vi "HEWH OSI Calculations.vi"(8 "Error In":errorcluster, 11 "Pressure Adjusted in":T1) -> (0 "Error Out":errorcluster, 1 "Power (Watts)":dbl, 2 "Current (Amps)":dbl, 3 "Pressure Adjusted out":T1, 4 "Voltage (Volts)":dbl)   [LabVIEW 2016]
uses:
  Type Definitions/HEWH MW100 Data Cluster.ctl
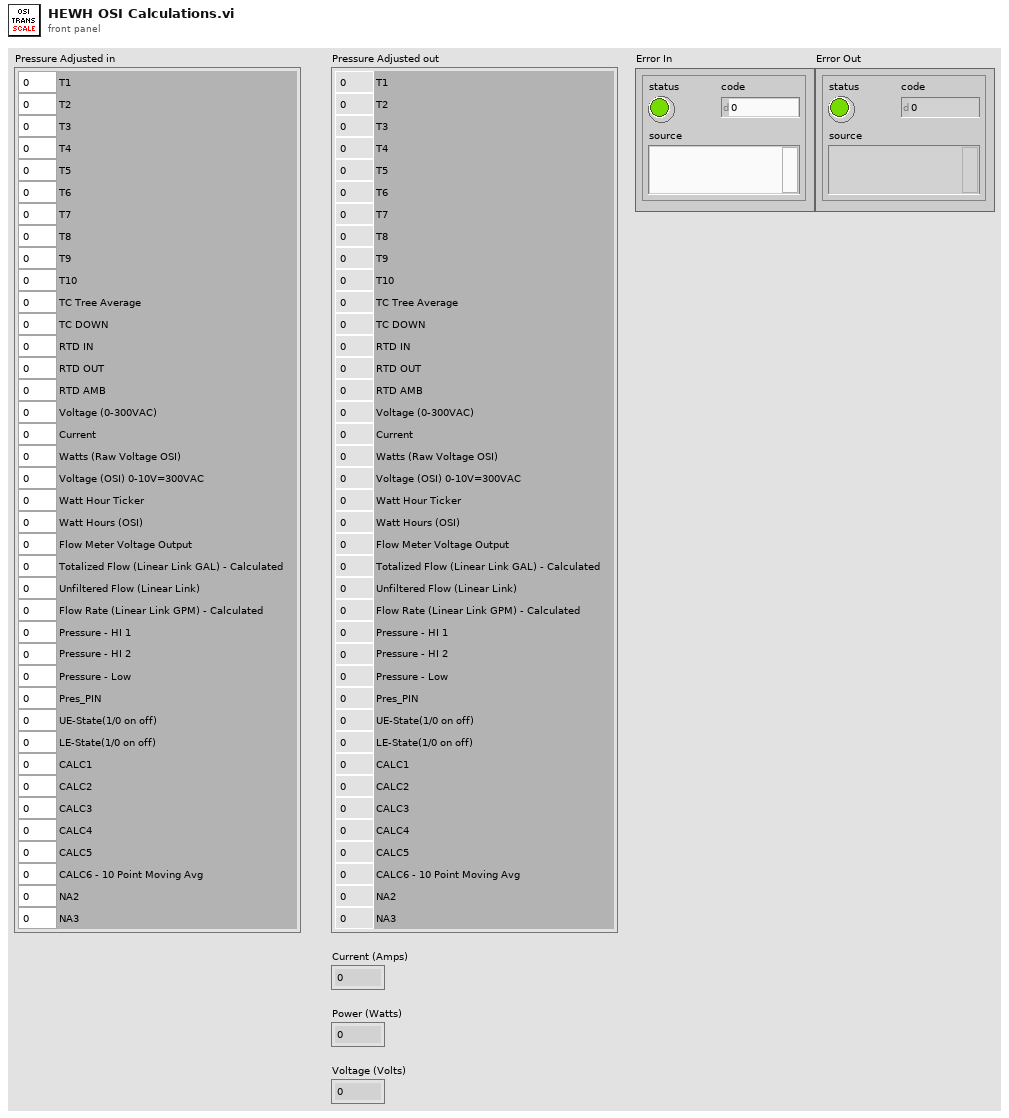
[diagram p1: front panel]
types:
  T1 = typedef "HEWH MW100 Data Cluster.ctl" = cluster{"T1":dbl, "T2":dbl, "T3":dbl, "T4":dbl, "T5":dbl, "T6":dbl, "T7":dbl, "T8":dbl, "T9":dbl, "T10":dbl, "TC Tree Average":dbl, "TC DOWN":dbl, "RTD IN":dbl, "RTD OUT":dbl, "RTD AMB":dbl, "Voltage (0-300VAC)":dbl, "Current":dbl, "Watts (Raw Voltage OSI)":dbl, "Voltage (OSI) 0-10V=300VAC":dbl, "Watt Hour Ticker":dbl, "Watt Hours (OSI)":dbl, "Flow Meter Voltage Output":dbl, "Totalized Flow (Linear Link GAL) - Calculated":dbl, "Unfiltered Flow (Linear Link)":dbl, "Flow Rate (Linear Link GPM) - Calculated":dbl, "Pressure - HI 1":dbl, "Pressure - HI 2":dbl, "Pressure - Low":dbl, "Pres_PIN":dbl, "UE-State(1/0 on off)":dbl, "LE-State(1/0 on off)":dbl, "CALC1":dbl, "CALC2":dbl, "CALC3":dbl, "CALC4":dbl, "CALC5":dbl, "CALC6 - 10 Point Moving Avg":dbl, "NA2":dbl, "NA3":dbl}
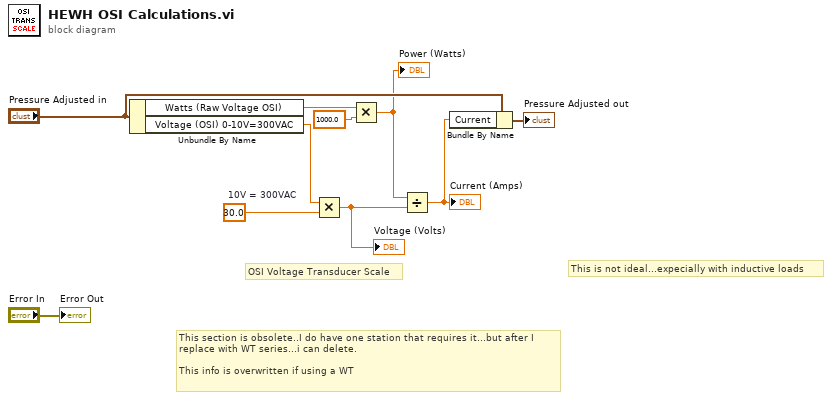
[diagram p0: block diagram]
diagram:
  w4 = 30.0  # 10V = 300VAC
  # "This is not ideal...expecially with inductive loads"
  # "This section is obsolete..I do have one station that requires it...but after I \nreplace with WT series...i can delete.\n\nThis info is overwritten if using a WT"
  # "OSI Voltage Transducer Scale"
  n1 = Unbundle By Name("Pressure Adjusted in") -> ("Watts (Raw Voltage OSI)"=w9:dbl, "Voltage (OSI) 0-10V=300VAC"=w10:dbl)
  n2 = Multiply(x=w10, y=w4) -> (x*y=w7:dbl)
  "Voltage (Volts)" <- w7
  n3 = Multiply(x=w9, y=1000.0) -> (x*y=w6:dbl)
  "Power (Watts)" <- w6
  n4 = Divide(x=w6, y=w7) -> (x/y=w5:dbl)
  "Current (Amps)" <- w5
  n5 = Bundle By Name(cluster="Pressure Adjusted in", "Current"=w5) -> (→"Pressure Adjusted out":T1)
  "Error Out" <- "Error In"
